vi "deleteSelectedFromRunDir.vi"(8 "error in (no error)":errorcluster, 11 "ExperimentRunner in":refnum<class "ExperimentRunner.lvclass">) -> (0 "error out":errorcluster, 3 "ExperimentRunner out":refnum<class "ExperimentRunner.lvclass">)   [LabVIEW 2011, in "Views.lvlib" / "ExperimentControl.lvlib" / "ExperimentRunner.lvclass"]
doc: "Delete the selected script from run directory"
uses:
  ExperimentRunner.lvclass
  ExperimentRunner.lvclass/ExperimentRunner.ctl
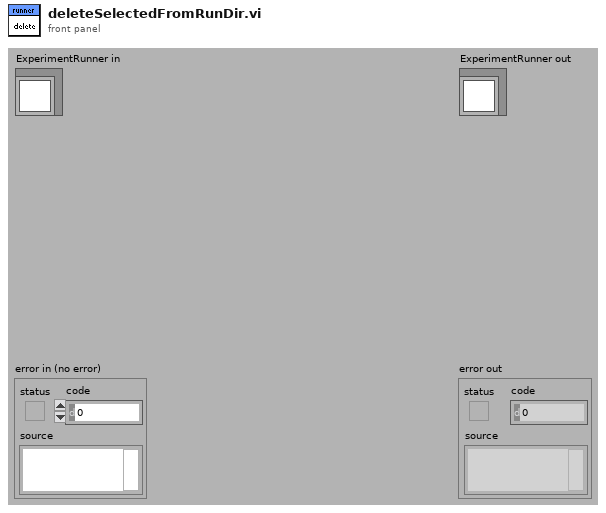
[diagram p1: front panel]
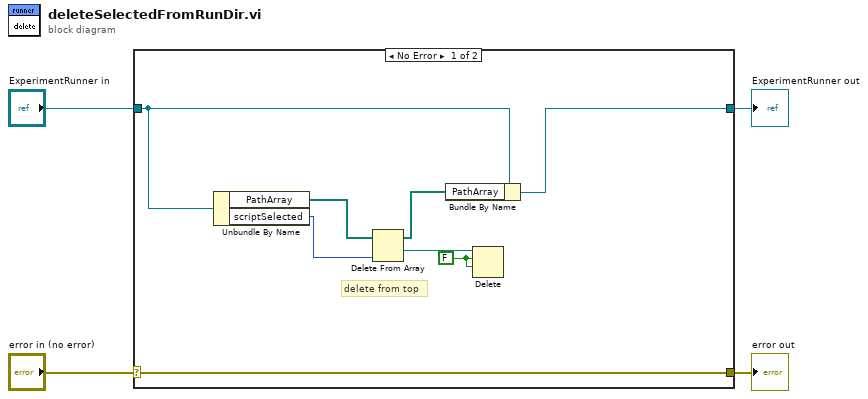
[diagram p0: block diagram]
diagram:
  n1 = case shown="No Error" "error in (no error)" {
    selector: "error in (no error)" -> [w12 w14]
    tunnel: [w12 w14] -> w3
    tunnel: [w7 w13] -> w1
    tunnel: "ExperimentRunner in" -> [w8 w13]
    frame No Error {
      w9 = FALSE ("entire hierarchy (F)")
      # "delete from top"
      n2 = Unbundle By Name(w8) -> ("PathArray"=w11:path[], "scriptSelected"=w5:i32)
      n3 = Delete From Array(array=w11, index=w5) -> (deleted portion=w10:path, array with subset deleted=w6:path[])  [unwired: 1 in]
      n4 = Bundle By Name(cluster=w8, "PathArray"=w6) -> (w7:refnum<class "ExperimentRunner.lvclass">)
      n5 = Delete(path (use dialog)=w10, entire hierarchy (F)=w9, confirm (F)=w9) -> ()  [unwired: 2 in, 3 out]
    }
    frame Error {
    }
  }
  "error out" <- w3
  "ExperimentRunner out" <- w1
